vi "Rx Section Page.vi"(8 "error in (no error)":errorcluster, 11 "Node Ptr":T1 format="%.0x") -> (0 "error out":errorcluster)   [LabVIEW 2019, in "UDP-Custom-Device System Explorer.lvlib"]
uses:
  UDP-Custom-Device System Explorer.lvlib
  <vilib>/NI VeriStand/Custom Device API/Custom Device Item Ref.ctl
  <vilib>/NI VeriStand/Custom Device API/Custom Device API.lvlib
  Property Accessors/Shared Section Accessors.lvlib
panel:
  in  "Rx Packets":i32[](listbox)
  in  "SHDocVw.IWebBrowser":refnum<k7>(container)
  in  "General Header":cluster{"Section Name":string}={"Section Name"="Configured Packets"}
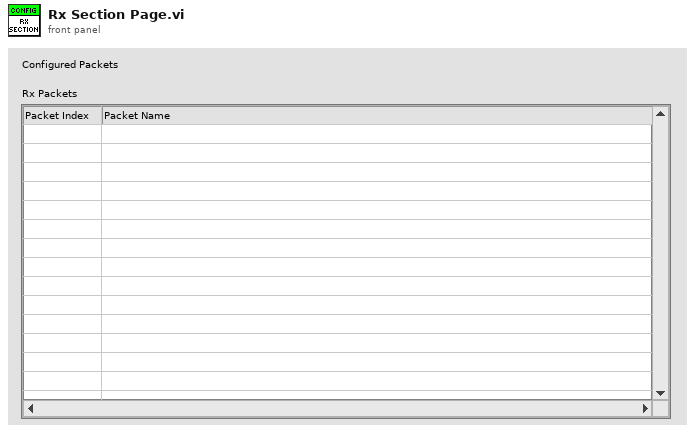
[diagram p1: front panel]
types:
  T1 = typedef "Custom Device API.lvlib/Custom Device Item Ref.ctl" = u64
  T2 = typedef "Custom Device API.lvlib/Custom Device Commands.ctl" = enum16{"Default", "Item renamed", "Shutdown", "Dynamic button pressed"}
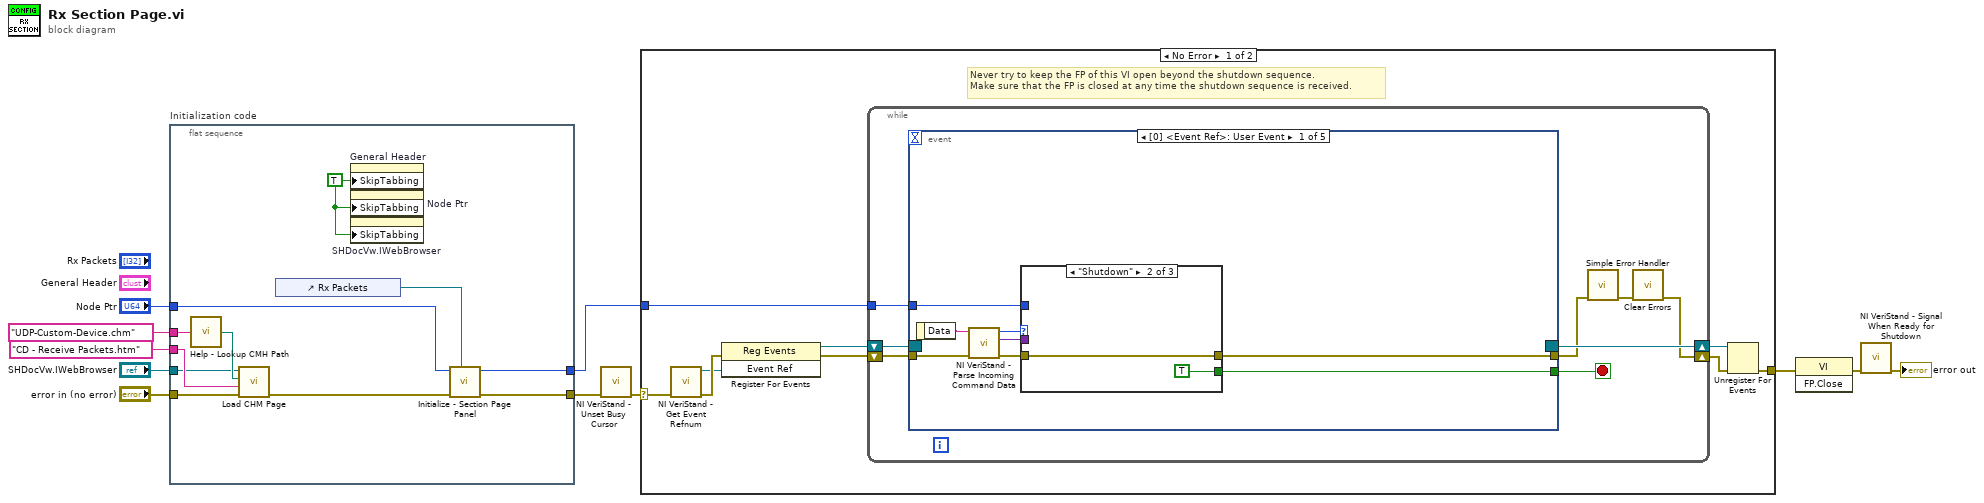
[diagram p0: block diagram]
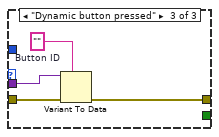
[diagram p3: hidden frame]
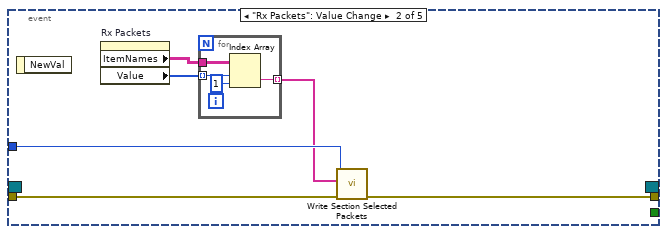
[diagram p4: hidden frame]
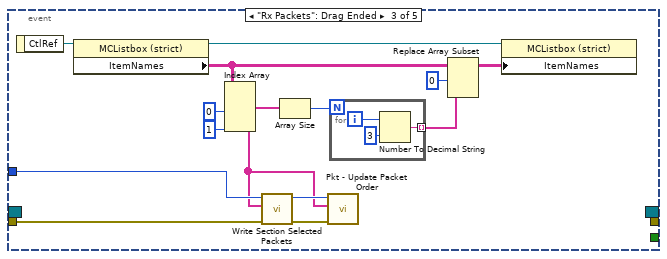
[diagram p5: hidden frame]
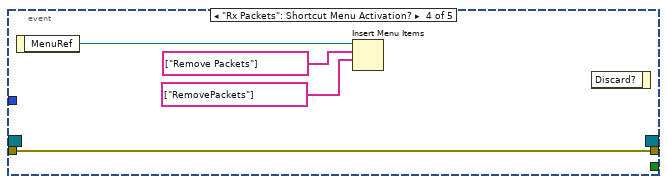
[diagram p6: hidden frame]
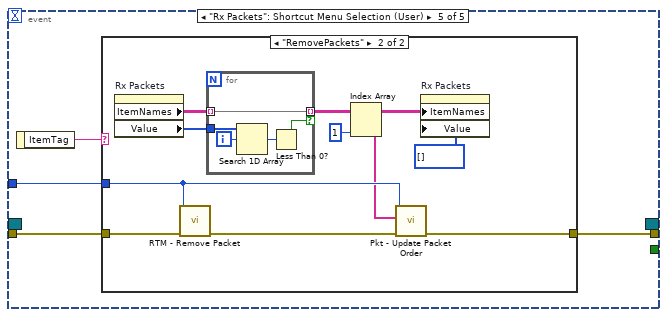
[diagram p7: hidden frame]
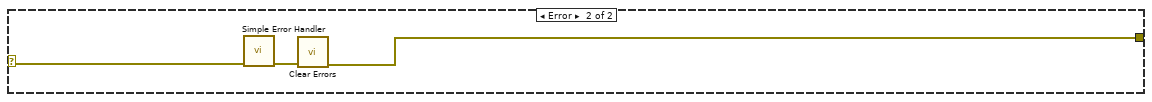
[diagram p9: hidden frame]
diagram:
  n1 = flat-sequence "Initialization code" {
    tunnel: "error in (no error)" -> [w18]
    tunnel: "Node Ptr" -> [w21]
    tunnel: [w22] -> w8
    tunnel: [w20] -> w5
    tunnel: "SHDocVw.IWebBrowser" -> [w15]
    tunnel: "CD - Receive Packets.htm" ("CD_CHM_Section") -> [w16]
    tunnel: "UDP-Custom-Device.chm" ("CD_CHM_FileName") -> [w17]
    frame #0 {
      w12 = TRUE ("Skip When Tabbing")
      n2 = call "Help - Lookup CMH Path.vi"("Main CMH File"=w17) -> ("Compiled CMH Path"=w19:path)
      n3 = call <vilib>:"Load CHM Page.vi"("error in (no error)"=w18, "HTML File"=w16, "Compiled CHM Path"=w19, "Web Browser Reference"=w15) -> ("error out"=w14:errorcluster)  [unwired: 7 in]
      n4 = control-ref of="Rx Packets"() -> (w13:refnum<vi>)
      n5 = property on="General Header" class="Clust (strict)"("SkipTabbing"=w12) -> ()  [unwired: 2 in, 2 out]
      n6 = property on="Node Ptr" class="DigNum (strict)"("SkipTabbing"=w12) -> ()  [unwired: 2 in, 2 out]
      n7 = property on="SHDocVw.IWebBrowser" class="AXCont"("SkipTabbing"=w12) -> ()  [unwired: 2 in, 2 out]
      n8 = call "Initialize - Section Page Panel.vi"("Packets Listbox"=w13, "error in (no error)"=w14, "Item Ref in"=w21) -> ("error out"=w22:errorcluster, "Item Ref out"=w20:T1)  [unwired: 7 in]
    }
  }
  n9 = call <vilib>:"NI VeriStand - Unset Busy Cursor.vi"("error in (no error)"=w8) -> ("error out"=w7:errorcluster)  [unwired: 10 out]
  n10 = case shown="No Error" w7 {
    selector: w7 -> [w23 w109]
    tunnel: [w28 w107] -> w11
    tunnel: w5 -> [w24 _]
    frame No Error {
      # "Never try to keep the FP of this VI open beyond the shutdown sequence.\nMake sure that the FP is closed at any time the shutdown sequence is received."
      n11 = call <vilib>:"NI VeriStand - Get Event Refnum.vi"("error in (no error)"=w23) -> ("error out"=w31:errorcluster, "Event Ref"=w27:refnum<user-event>)  [unwired: 9 out]
      n12 = register-events(error in=w31, w27) -> (reference out=w25:refnum<event-registration>, error out=w26:errorcluster)  [unwired: 1 in]
      n13 = while {
        tunnel: w24 -> [w35]
        shift-right: [w32] -> w29
        shift-left: w26 -> [w38]
        shift-right: [w39] -> w30
        shift-left: w25 -> [w37]
        stop <- w36 stop-if-true
        n14 = event shown="[0] <Event Ref>: User Event" {
          selector: w37 -> [_ _ _ _ _]
          dyn-events: [_ _ _ _ _] -> w39
          timeout: _ -> [_ _ _ _ _]
          tunnel: w38 -> [w47 w56 w70 w83 w90]
          tunnel: [w43 _ _ _ _] -> w36
          tunnel: [w42 w55 _ w83 w87] -> w34
          tunnel: w35 -> [w41 w58 w72 _ w88]
          event User Event {
            n15 = event-data() -> ("Data"=w46:string)  [unwired: 1 out]
            n16 = call <vilib>:"NI VeriStand - Parse Incoming Command Data.vi"("error in (no error)"=w47, "Incoming data"=w46) -> ("error out"=w45:errorcluster, "Outgoing data"=w40:variant, "Action"=w44:T2)  [unwired: 7 out]
            n17 = case shown="\"Shutdown\"" w44 {
              tunnel: w45 -> [w48 w49 w54]
              tunnel: [_ TRUE _] -> w43
              tunnel: [w48 w49 w51] -> w42
              tunnel: w41 -> [_ _ _]
              tunnel: w40 -> [_ _ w53]
              frame "Default", Default {
              }
              frame "Shutdown" {
              }
              frame "Dynamic button pressed" {
                w52 = ""  # Button ID
                n18 = Variant To Data(error in=w54, type=w52, Variant=w53) -> (error out=w51:errorcluster)  [unwired: 1 out]
              }
            }
          }
          event "Rx Packets": Value Change {
            n19 = event-data() -> ()  [unwired: 2 out]
            n20 = property on="Rx Packets" class="MCListbox (strict)"() -> ("ItemNames"=w59:string[][], "Value"=w60:i32[])  [unwired: 2 in, 2 out]
            n21 = for {
              tunnel: w59 -> [w64]
              tunnel: [w63] -> w57 mode=indexing
              tunnel: w60 -> [w62] mode=indexing
              n22 = Index Array(array=w64, index (row)=w62, index (col)=1 ("disabled index (row)")) -> (element=w63:string)
            }
            n23 = call "Write Section Selected Packets.vi"("error in (no error)"=w56, "Selected Packets"=w57, "Node Ptr"=w58) -> ("error out"=w55:errorcluster)  [unwired: 7 in, 1 out]
          }
          event "Rx Packets": Drag Ended {
            n24 = event-data() -> ("CtlRef"=w68:refnum<vi>)  [unwired: 1 out]
            n25 = property class="MCListbox (strict)"(reference=w68) -> (reference out=w67:refnum<vi>, "ItemNames"=w79:string[][])  [unwired: 1 in, 1 out]
            n26 = Index Array(array=w79, index (col) #1=0 ("disabled index (col)"), index (col) #2=1 ("index (col)")) -> (element #1=w75:string[], element #2=w65:string[])  [unwired: 2 in]
            n27 = call "Write Section Selected Packets.vi"("error in (no error)"=w70, "Selected Packets"=w65, "Node Ptr"=w72) -> ("error out"=w69:errorcluster, "Node Ptr out"=w71:T1)  [unwired: 7 in]
            n28 = Array Size(array=w75) -> (size(s)=w76:i32)
            n29 = call "Pkt - Update Packet Order.vi"("error in (no error)"=w69, "Channel Names"=w65, "Node Ptr"=w71) -> ()  [unwired: 7 in, 2 out]
            n30 = for {
              N: w76 -> [_]
              tunnel: [w80] -> w78 mode=indexing
              i -> [w82]
              n31 = Number To Decimal String(number=w82, width (-)=i16 3) -> (decimal integer string=w80:string)
            }
            n32 = Replace Array Subset(array=w79, new element=w78, index (col)=0 ("disabled index (col)")) -> (w73:string[][])  [unwired: 1 in]
            n33 = property class="MCListbox (strict)"(reference=w67, "ItemNames"=w73) -> ()  [unwired: 1 in, 2 out]
          }
          event "Rx Packets": Shortcut Menu Activation? {
            n34 = event-data() -> ("MenuRef"=w84:refnum<k9>)  [unwired: 1 out]
            n35 = Insert Menu Items(7:string[] ["RemovePackets"] ("item names"), 8:string[] ["Remove Packets"] ("item names"), 9:w84) -> ()  [unwired: 3 in, 3 out]
            n36 = event-data() -> ()  [unwired: 2 in, 1 out]
          }
          event "Rx Packets": Shortcut Menu Selection (User) {
            n37 = event-data() -> ("ItemTag"=w89:string)  [unwired: 1 out]
            n38 = case shown="\"RemovePackets\"" w89 {
              tunnel: w90 -> [w91 w101]
              tunnel: w88 -> [_ w97]
              tunnel: [w91 w96] -> w87
              frame Default {
              }
              frame "RemovePackets" {
                n39 = property on="Rx Packets" class="MCListbox (strict)"() -> ("ItemNames"=w100:string[][], "Value"=w99:i32[])  [unwired: 2 in, 2 out]
                n40 = call "RTM - Remove Packet.vi"("error in (no error)"=w101, "Node Ptr"=w97) -> ("error out"=w94:errorcluster)  [unwired: 9 in]
                n41 = for {
                  tunnel: w99 -> [w105]
                  tunnel: [w106] -> w93 mode=indexing if=w102
                  tunnel: w100 -> [w106] mode=indexing
                  i -> [w104]
                  n42 = Search 1D Array(1D array=w105, element=w104) -> (index of element=w103:i32)  [unwired: 1 in]
                  n43 = Less Than 0?(x=w103) -> (x < 0?=w102:bool)
                }
                n44 = Index Array(array=w93, index (col)=1 ("disabled index (col)")) -> (element=w92:string[])  [unwired: 1 in]
                n45 = call "Pkt - Update Packet Order.vi"("error in (no error)"=w94, "Channel Names"=w92, "Node Ptr"=w97) -> ("error out"=w96:errorcluster)  [unwired: 7 in, 1 out]
                n46 = property on="Rx Packets" class="MCListbox (strict)"("ItemNames"=w93, "Value"=i32[] [] ("Rx Packets")) -> ()  [unwired: 2 in, 2 out]
              }
            }
          }
        }
        n47 = call <vilib>:"Simple Error Handler.vi"("error in (no error)"=w34) -> ("error out"=w33:errorcluster)  [unwired: 1 in, 7 out]
        n48 = call <vilib>:"Clear Errors.vi"("error in (no error)"=w33) -> ("error out"=w32:errorcluster)  [unwired: 1 in, 5 out]
      }
      n49 = Unregister For Events(event registration refnum=w30, error in=w29) -> (error out=w28:errorcluster)
    }
    frame Error {
      n50 = call <vilib>:"Simple Error Handler.vi"("error in (no error)"=w109) -> ("error out"=w108:errorcluster)  [unwired: 1 in, 7 out]
      n51 = call <vilib>:"Clear Errors.vi"("error in (no error)"=w108) -> ("error out"=w107:errorcluster)  [unwired: 1 in, 5 out]
    }
  }
  n52 = invoke class="VI" method="FP.Close"(error in=w11) -> (error out=w10:errorcluster)  [unwired: 2 in, 2 out]
  n53 = call <vilib>:"NI VeriStand - Signal When Ready for Shutdown.vi"("error in (no error)"=w10) -> ("error out"=→"error out":errorcluster)  [unwired: 10 out]
